vi "MatchInputs.vi"(7 "type to match":variant, 8 "error in":errorcluster, 11 "Inputs":variant) -> (0 "error out":errorcluster, 1 "Matched?":bool, 3 "Matched Inputs":variant[](array[variant]))   [LabVIEW 2021, in "smo.lvlib"]
uses:
  smo.lvlib
  <vilib>/Utility/VariantDataType/Type.ctl
  <vilib>/Utility/VariantDataType/VariantType.lvlib
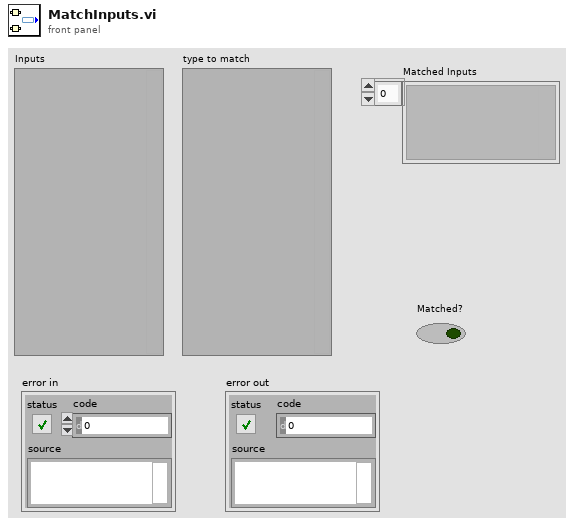
[diagram p1: front panel]
types:
  T1 = typedef "VariantType.lvlib/Type.ctl" = enum8{"Invalid Type", "Void", "I8", "I16", "I32", "I64", "U8", "U16", "U32", "U64", "Single Float", "Double Float", "Extended Float", "Single Complex", "Double Complex", "Extended Complex", "Enum U8", "Enum U16", "Enum U32", "Enum U64", "Single Float With Unit", "Double Float With Unit", "Extended Float With Unit", "Single Complex with Unit", "Double Complex with Unit", "Extended Complex with Unit", "Boolean", "String", "Path", "Picture", "Tag", "Array", "Cluster", "Variant", "LV Variant", "Waveform", "Timestamp", "Digital Waveform", "Digital Data", "ExpressData", "Refnum", "External Data", "VI", "Poly VI", "LabVIEW Class Instance", "Fixed Point"}
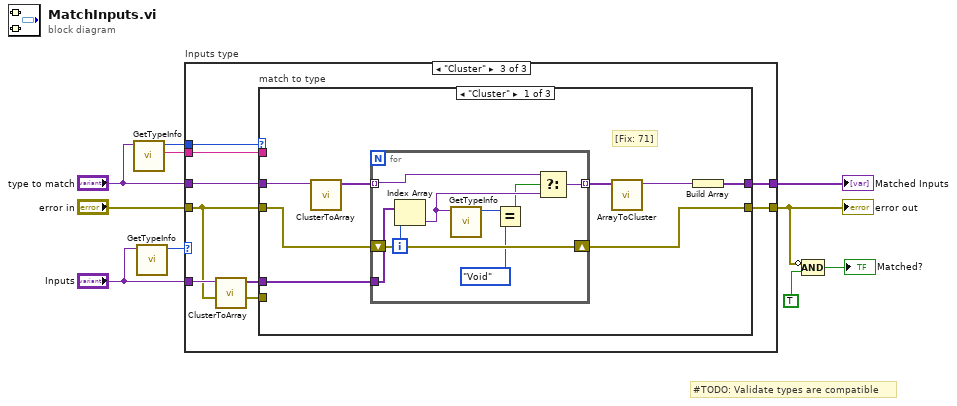
[diagram p0: block diagram]
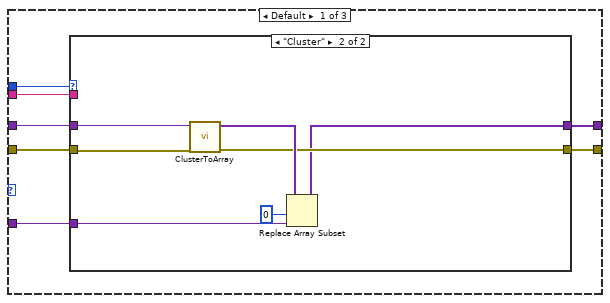
[diagram p2: hidden frame]
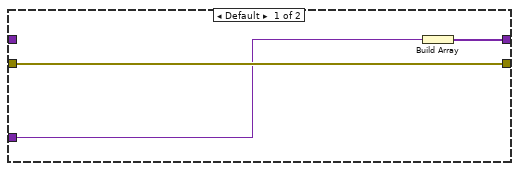
[diagram p3: hidden frame]
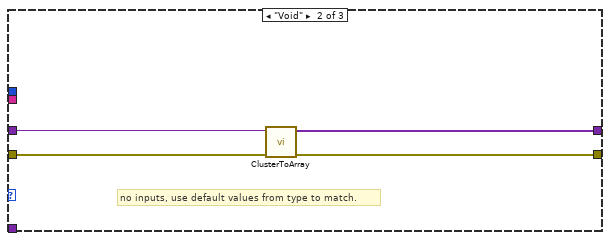
[diagram p4: hidden frame]
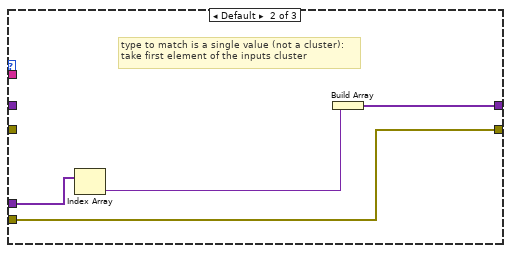
[diagram p5: hidden frame]
diagram:
  # "#TODO: Validate types are compatible"
  n1 = call <vilib>:"GetTypeInfo.vi"("Variant"="type to match") -> ("Name"=w6:string, "Type Enum"=w7:T1)  [unwired: 6 in, 3 out]
  n2 = call <vilib>:"GetTypeInfo.vi"("Variant"="Inputs") -> ("Type Enum"=w4:T1)  [unwired: 6 in, 4 out]
  n3 = case "Inputs type" shown="\"Cluster\"" w4 {
    tunnel: "Inputs" -> [w17 _ w32]
    tunnel: "type to match" -> [w16 w28 w37]
    tunnel: [w15 w27 w36] -> w9
    tunnel: "error in" -> [w14 w29 w30]
    tunnel: [w13 w29 w35] -> w3
    tunnel: w7 -> [w12 _ w34]
    tunnel: w6 -> [w11 _ w33]
    frame Default {
      n4 = case shown="\"Cluster\"" w12 {
        tunnel: w17 -> [w18 w25]
        tunnel: w16 -> [_ w24]
        tunnel: [w20 w21] -> w15
        tunnel: w14 -> [w19 w22]
        tunnel: [w19 w22] -> w13
        tunnel: w11 -> [_ _]
        frame Default {
          n5 = Build Array(w18) -> (w20:variant[])
        }
        frame "Cluster" {
          n6 = call "ClusterToArray.vi"("Cluster"=w24) -> ("Array"=w23:variant[])  [unwired: 10 in]
          n7 = Replace Array Subset(array=w23, new element=w25, index=0) -> (w21:variant[])
        }
      }
    }
    frame "Void" {
      # "no inputs, use default values from type to match."
      n8 = call "ClusterToArray.vi"("Cluster"=w28) -> ("Array"=w27:variant[])  [unwired: 10 in]
    }
    frame "Cluster" {
      n9 = call "ClusterToArray.vi"("Cluster"=w32) -> ("Array"=w31:variant[])  [unwired: 10 in]
      n10 = case "match to type" shown="\"Cluster\"" w34 {
        tunnel: w37 -> [w44 _ _]
        tunnel: [w40 w57 _] -> w36
        tunnel: [w42 w56 w59] -> w35
        tunnel: w31 -> [w45 w58 _]
        tunnel: w30 -> [_ w56 _]
        tunnel: w30 -> [w41 _ w59]
        tunnel: w33 -> [_ _ _]
        frame "Cluster" {
          # "[Fix: 71]"
          n11 = call "ClusterToArray.vi"("Cluster"=w44) -> ("Array"=w43:variant[])  [unwired: 10 in]
          n12 = for {
            shift-right: [w52] -> w42
            shift-left: w41 -> [w52]
            tunnel: w43 -> [w51] mode=indexing
            tunnel: [w49] -> w39 mode=indexing
            tunnel: w45 -> [w53]
            i -> [w54]
            n13 = Index Array(array=w53, index=w54) -> (element=w50:variant)
            n14 = call <vilib>:"GetTypeInfo.vi"("Variant"=w50) -> ("Type Enum"=w48:T1)  [unwired: 6 in, 4 out]
            n15 = Equal?(x=w48, y=Type."Void") -> (x = y?=w46:bool)
            n16 = Select(t=w51, s=w46, f=w50) -> (s? t:f=w49:variant)
          }
          n17 = call "ArrayToCluster.vi"("Array"=w39) -> ("Cluster"=w38:variant)  [unwired: 10 in]
          n18 = Build Array(w38) -> (w40:variant[])
        }
        frame Default {
          # "type to match is a single value (not a cluster):\ntake first element of the inputs cluster"
          n19 = Index Array(array=w58) -> (element=w55:variant)  [unwired: 1 in]
          n20 = Build Array(w55) -> (w57:variant[])
        }
        frame "Void" {
        }
      }
    }
  }
  "error out" <- w3
  "Matched Inputs" <- w9
  n21 = Compound Arithmetic op=AND(invert w3, TRUE) -> (→"Matched?":bool)
